vi "Material-Line 1-Normalize.vi"(8 "error in (no error)":errorcluster, 11 "Material-RunTest in":refnum<class "Material-RunTest.lvclass">) -> (0 "error out":errorcluster, 3 "Material-RunTest out":refnum<class "Material-RunTest.lvclass">)   [LabVIEW 2013, in "Material-RunTest.lvclass"]
uses:
  Material-RunTest.lvclass
  Material-RunTest.lvclass/Material-RunTest.ctl
  <userlib>/_MGI/1D Array/MGI Average/MGI Average (DBL[]).vi
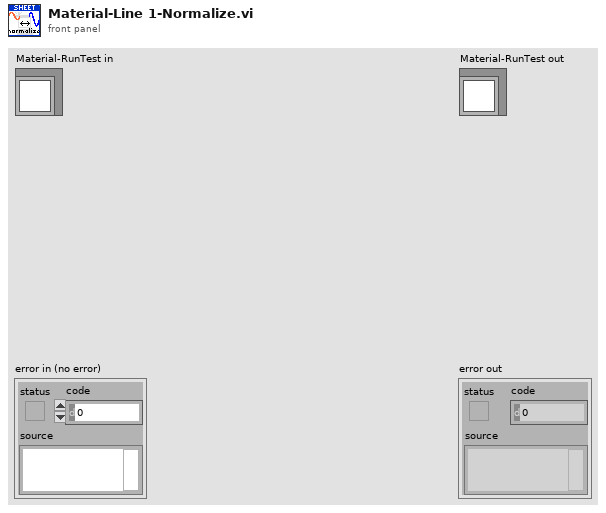
[diagram p1: front panel]
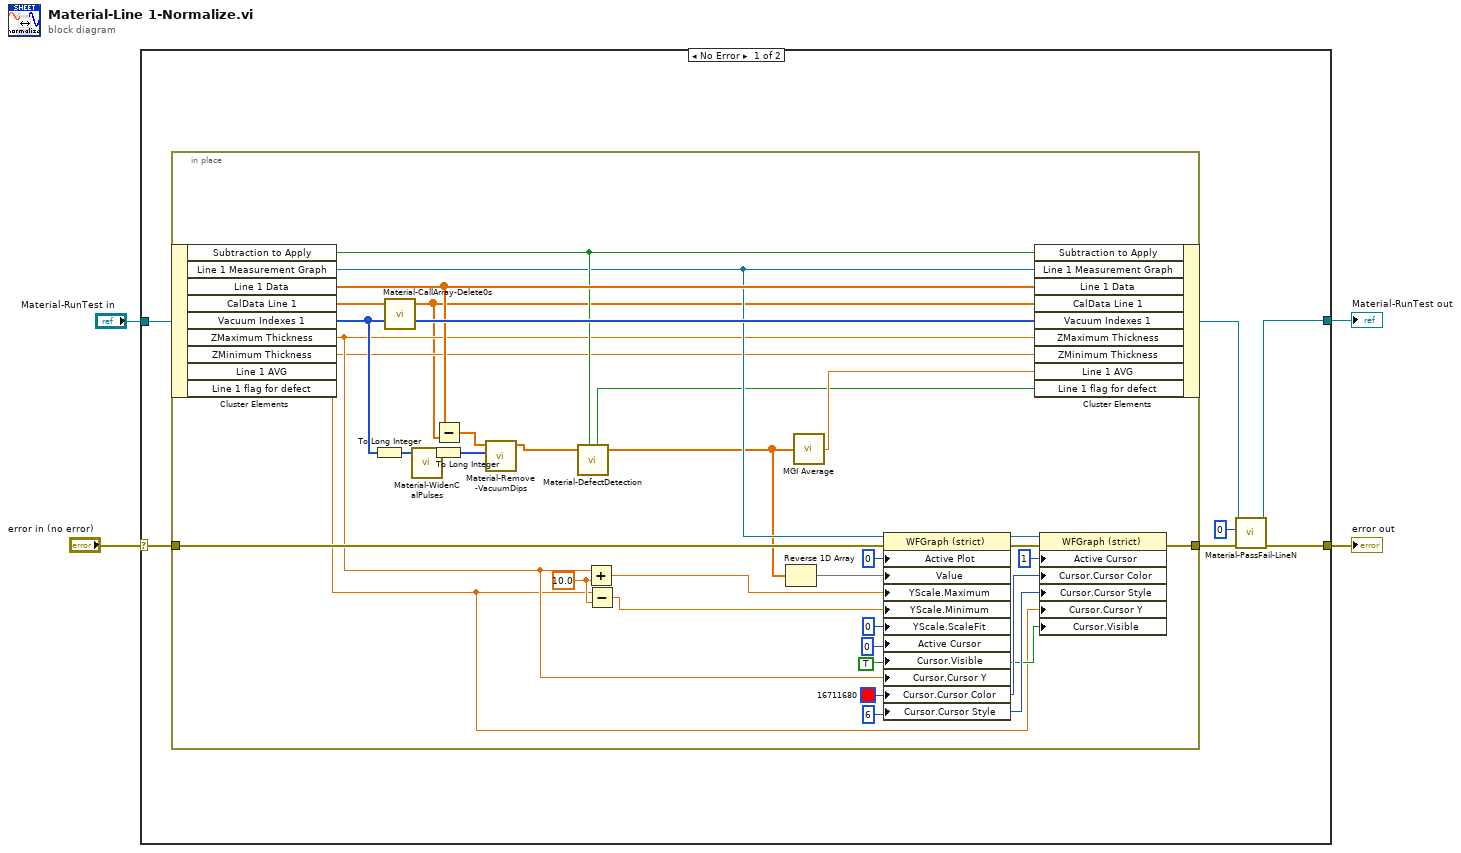
[diagram p0: block diagram]
diagram:
  n1 = case shown="No Error" "error in (no error)" {
    selector: "error in (no error)" -> [w10 w44]
    tunnel: [w7 w44] -> w3
    tunnel: [w5 w43] -> w1
    tunnel: "Material-RunTest in" -> [w11 w43]
    frame No Error {
      n2 = in-place {
        in-place-border: w10 -> [w30]
        in-place-border: [w23] -> w9
        w26 = u32 16711680
        w25 = u8 6 ("Cursor.Cursor Style")
        w36 = 10.0 ("y")
        w24 = TRUE ("Cursor.Visible")
        n3 = in-place-cluster #1(w11) -> ("Subtraction to Apply"=w33:bool, "Line 1 Measurement Graph"=w32:refnum<vi>, "Line 1 Data"=w34:dbl[], "CalData Line 1"=w15:dbl[], "Vacuum Indexes 1"=w35:i32[], "ZMaximum Thickness"=w19:dbl, "ZMinimum Thickness"=w18:dbl)  [unwired: 2 out]
        n4 = To Long Integer(number=w35) -> (32bit integer=w39:i32[])
        n5 = call "Material-CallArray-Delete0s.vi"("CalData Line 3"=w15) -> ("array w/ subset deleted"=w14:dbl[])  [unwired: 8 in]
        n6 = call "Material-WidenCalPulses.vi"("raw CAL indexes"=w39) -> ("New Indexes"=w41:u32[])  [unwired: 8 in]
        n7 = To Long Integer(number=w41) -> (32bit integer=w42:i32[])
        n8 = Subtract(x=w34, y=w14) -> (x-y=w40:dbl[])
        n9 = call "Material-Remove-VacuumDips.vi"("input array of indexes"=w42, "Input Data"=w40) -> ("Conditioned output"=w37:dbl[])  [unwired: 9 in]
        n10 = call "Material-DefectDetection.vi"("Conditioned output"=w37, "Subtraction to Apply"=w33) -> ("Flagged for Defect"=w22:bool, "Array"=w13:dbl[])  [unwired: 6 in]
        n11 = Add(x=w19, y=w36) -> (x+y=w21:dbl)
        n12 = Subtract(x=w18, y=w36) -> (x-y=w20:dbl)
        n13 = Reverse 1D Array(array=w13) -> (reversed array=w12:dbl[])
        n14 = call-poly <userlib>:"MGI Average.vi"("Double[]"=w13) -> ("Average"=w31:dbl)  [unwired: 1 in]
        n15 = property class="WFGraph (strict)"(reference=w32, error in=w30, "Active Plot"=u32 0, "Value"=w12, "YScale.Maximum"=w21, "YScale.Minimum"=w20, "YScale.ScaleFit"=u8 0 ("Y Scale.Scale Fit"), "Active Cursor"=u32 0, "Cursor.Visible"=w24, "Cursor.Cursor Y"=w19, "Cursor.Cursor Color"=w26, "Cursor.Cursor Style"=w25) -> (reference out=w28:refnum<vi>, error out=w29:errorcluster)
        n16 = in-place-cluster #1("Subtraction to Apply"=w33, "Line 1 Measurement Graph"=w32, "Line 1 Data"=w34, "CalData Line 1"=w14, "Vacuum Indexes 1"=w35, "ZMaximum Thickness"=w19, "ZMinimum Thickness"=w18, "Line 1 AVG"=w31, "Line 1 flag for defect"=w22) -> (w6:refnum<class "Material-RunTest.lvclass">)
        n17 = property class="WFGraph (strict)"(reference=w28, error in=w29, "Active Cursor"=u32 1, "Cursor.Cursor Color"=w26, "Cursor.Cursor Style"=w25, "Cursor.Cursor Y"=w18, "Cursor.Visible"=w24) -> (error out=w23:errorcluster)  [unwired: 1 out]
      }
      n18 = call "Material-PassFail-LineN.vi"("error in (no error)"=w9, "Line?"=0, "Material-RunTest in"=w6) -> ("error out"=w7:errorcluster, "Material-RunTest out"=w5:refnum<class "Material-RunTest.lvclass">)  [unwired: 7 in]
    }
    frame Error {
    }
  }
  "error out" <- w3
  "Material-RunTest out" <- w1
